vi "Gender_Age_Hight.vi"(9 "Gender":enum32{"Male", "Female"}(radio), 10 "height":dbl, 11 "age":dbl) -> (3 "Dataset":i32[](array[numeric]))   [LabVIEW 2023]
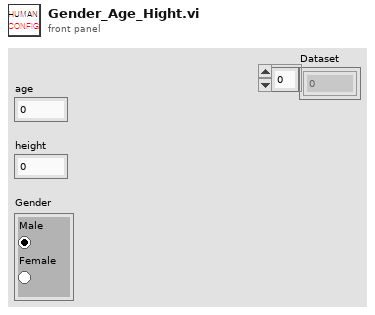
[diagram p1: front panel]
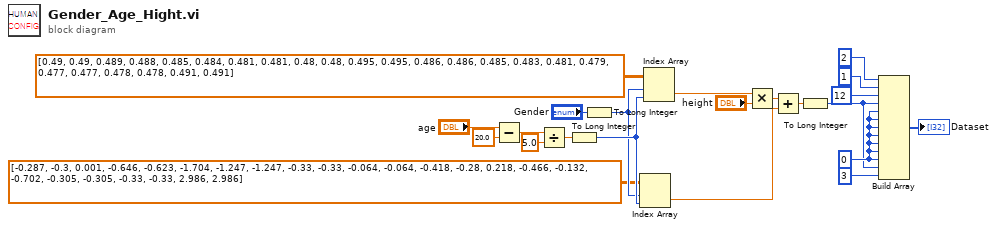
[diagram p0: block diagram]
diagram:
  w4 = 0 ("원소")
  n1 = Subtract(x="age", y=20.0) -> (x-y=w13:dbl)
  n2 = Divide ("나누기")(x=w13, y=5.0) -> (x/y=w15:dbl)
  n3 = To Long Integer(number=w15) -> (32bit integer=w18:i32)
  n4 = To Long Integer(number="Gender") -> (32bit integer=w17:i32)
  n5 = Index Array(array=dbl[][] [[-0.287, -0.3, 0.001, -0.646, -0.623, -1.704, -1.247, -1.247, -0.33, -0.33, -0.064, -0.064], [-0.418, -0.28, 0.218, -0.466, -0.132, -0.702, -0.305, -0.305, -0.33, -0.33, 2.986, 2.986]], index (row)=w17, index (col)=w18) -> (element=w22:dbl)
  n6 = Index Array(array=dbl[][] [[0.49, 0.49, 0.489, 0.488, 0.485, 0.484, 0.481, 0.481, 0.48, 0.48, 0.495, 0.495], [0.486, 0.486, 0.485, 0.483, 0.481, 0.479, 0.477, 0.477, 0.478, 0.478, 0.491, 0.491]], index (row)=w17, index (col)=w18) -> (element=w19:dbl)
  n7 = Multiply(x=w19, y="height") -> (x*y=w21:dbl)
  n8 = Add(x=w21, y=w22) -> (x+y=w8:dbl)
  n9 = To Long Integer(number=w8) -> (32bit integer=w3:i32)
  n10 = Build Array(2, 1 ("원소"), 12 ("원소"), w3, w4, w4, w4, w4, w4, w4, w4, w3, 3 ("원소")) -> (→"Dataset":i32[])
